vi "Delete Data Attributes.vi"(8 "error in (no error)":errorcluster, 11 "Data.lvclass":refnum<class "Data.lvclass">) -> (0 "error out":errorcluster)   [LabVIEW 2017, in "Data.lvclass"]
uses:
  <vilib>/addons/_NISVFA/_Shared subVIs/Data Objects/Data/Data.lvclass
  <vilib>/addons/_NISVFA/_Shared subVIs/Data Objects/Data/Data.lvclass/Data.ctl
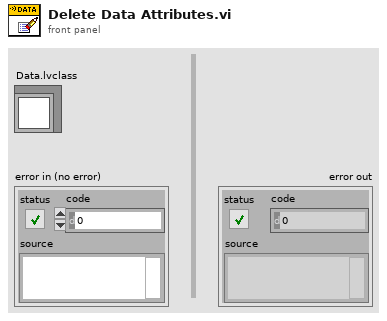
[diagram p1: front panel]
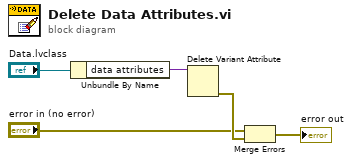
[diagram p0: block diagram]
diagram:
  n1 = Unbundle By Name("Data.lvclass") -> ("data attributes"=w4:variant)
  n2 = Delete Variant Attribute(7:w4) -> (0:w3:errorcluster)  [unwired: 2 in, 2 out]
  n3 = Merge Errors("error in (no error)", w3) -> (→"error out":errorcluster)
